vi "Init_PCAN.vi"(2 "type":i32, 3 "baud":u16) -> (0 "Boolean":bool, 1 "Version":string)   [LabVIEW 2017]
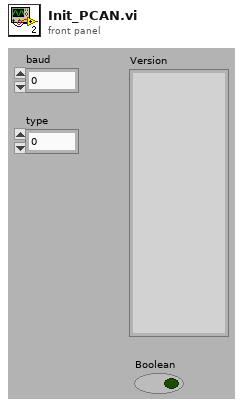
[diagram p1: front panel]
types:
  T1 = cluster{"Is Warning":bool, "Is Error":bool, "Message":string}
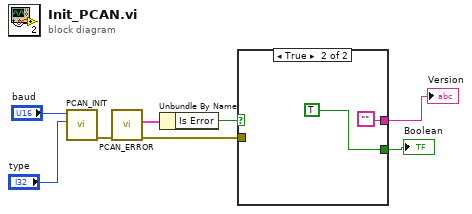
[diagram p0: block diagram]
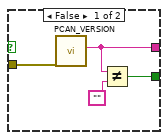
[diagram p2: hidden frame]
diagram:
  n1 = call "PCAN_INIT.vi"("Msg Type"="type", "BTR0BTR1"="baud") -> ("error out"=w4:errorcluster)  [unwired: 2 in, 7 out]
  n2 = call "PCAN_ERROR.vi"("error in (no error)"=w4) -> ("error out"=w7:errorcluster, "PCAN error"=w5:T1)  [unwired: 1 in, 8 out]
  n3 = Unbundle By Name(w5) -> ("Is Error"=w6:bool)
  n4 = case shown="True" w6 {
    tunnel: w7 -> [w12 _]
    tunnel: [w10 TRUE] -> w8
    tunnel: [w9 ""] -> w1
    frame False {
      n5 = call "PCAN_VERSION.vi"("error in (no error)"=w12) -> ("lpszTextBuff"=w9:string)  [unwired: 1 in, 9 out]
      n6 = Not Equal?(x=w9, y="") -> (x != y?=w10:bool)
    }
    frame True {
    }
  }
  "Boolean" <- w8
  "Version" <- w1
